vi "Lightning Begin.vi"() -> (0 "error out":errorcluster)   [LabVIEW 2015]
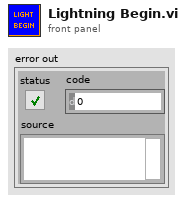
[diagram p1: front panel]
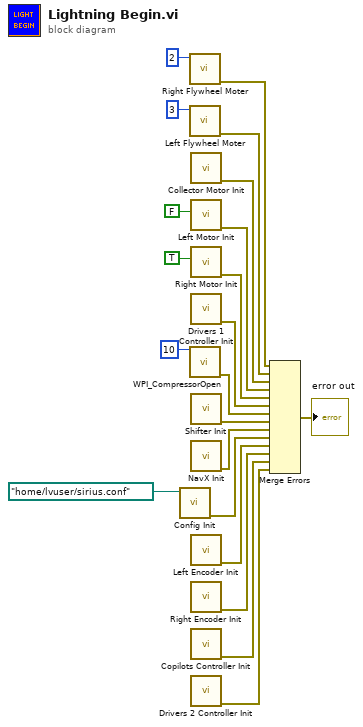
[diagram p0: block diagram]
diagram:
  n1 = call "Config Init.vi"("Path"=path "/home/lvuser/sirius.conf") -> ("error out"=w14:errorcluster)  [unwired: 10 in]
  n2 = call "Right Flywheel Moter.vi"("CAN Id"=u8 2) -> ("error out"=w5:errorcluster)  [unwired: 10 in]
  n3 = call "Left Flywheel Moter.vi"("CAN Id"=u8 3) -> ("error out"=w6:errorcluster)  [unwired: 10 in]
  n4 = call <vilib>:"WPI_CompressorOpen.vi"("Pneumatics Control Module (0)"=u8 10) -> ("error out"=w17:errorcluster)  [unwired: 13 in, 1 out]
  n5 = call "Collector Motor Init.vi"() -> ("error out"=w8:errorcluster)  [unwired: 11 in]
  n6 = call "Left Motor Init.vi"("Invert (default false)"=FALSE) -> ("error out"=w20:errorcluster)  [unwired: 10 in]
  n7 = call "Right Motor Init.vi"("Invert (default false)"=TRUE) -> ("error out"=w21:errorcluster)  [unwired: 10 in]
  n8 = call "Drivers 1 Controller Init.vi"() -> ("error out"=w18:errorcluster)  [unwired: 11 in]
  n9 = call "Shifter Init.vi"() -> ("Error Out"=w16:errorcluster)  [unwired: 11 in]
  n10 = call "NavX Init.vi"() -> ("error out"=w15:errorcluster)  [unwired: 11 in]
  n11 = call "Left Encoder Init.vi"() -> ("error out"=w12:errorcluster)  [unwired: 11 in]
  n12 = call "Right Encoder Init.vi"() -> ("error out"=w11:errorcluster)  [unwired: 11 in]
  n13 = call "Copilots Controller Init.vi"() -> ("error out"=w7:errorcluster)  [unwired: 11 in]
  n14 = call "Drivers 2 Controller Init.vi"() -> ("error out"=w1:errorcluster)  [unwired: 11 in]
  n15 = Merge Errors(w5, w6, w8, w20, w21, w18, w17, w16, w15, w14, w12, w11, w7, w1) -> (→"error out":errorcluster)
